vi "Colonoscopy competition - calcutate bias.vi"(11 "Potentiometer (V)":dbl) -> (3 "Bias (-1 to +1)":dbl)   [LabVIEW 2016]
uses:
  <vilib>/Analysis/3filter.llb/Filter Passband Type.ctl
  <vilib>/Analysis/NI_AALBase.lvlib
  <vilib>/ptbypt/NI_PtbyPt.lvlib
panel:
  # "Outputs"
  # "Inputs"
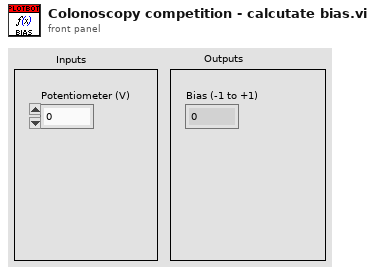
[diagram p1: front panel]
types:
  T1 = typedef "NI_AALBase.lvlib/Filter Passband Type.ctl" = enum32{"Lowpass", "Highpass", "Bandpass", "Bandstop"}
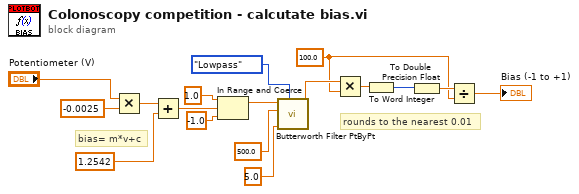
[diagram p0: block diagram]
diagram:
  w2 = 100.0 ("y")
  # "rounds to the nearest 0.01"
  # "bias= m*v+c"
  n1 = Multiply(x="Potentiometer (V)", y=-0.0025) -> (x*y=w17:dbl)
  n2 = Add(x=w17, y=1.2542) -> (x+y=w13:dbl)
  n3 = In Range and Coerce(upper limit=1.0 ("x"), x=w13, lower limit=-1.0) -> (coerced(x)=w10:dbl)  [unwired: 1 out]
  n4 = call <vilib>:"Butterworth Filter PtByPt.vi"("filter type"=Filter_Passband_Type."Lowpass", "low cutoff freq: fl"=5.0 ("high cutoff freq: fh"), "sampling freq: fs"=500.0, "x"=w10) -> ("Filtered x"=w6:dbl)  [unwired: 5 in, 1 out]
  n5 = Multiply(x=w6, y=w2) -> (x*y=w5:dbl)
  n6 = To Word Integer(number=w5) -> (16bit integer=w4:i16)
  n7 = To Double Precision Float(number=w4) -> (double precision float=w3:dbl)
  n8 = Divide(x=w3, y=w2) -> (x/y=→"Bias (-1 to +1)":dbl)
